vi "Follower SetControl.vi"(0 "DeviceReference":T1, 1 "StopSendingOtherRequests":bool=TRUE, 2 "MasterID":i32, 3 "OpposeMasterDirection":bool, 7 "error in":errorcluster, 18 "Update Frequency (Hz)":dbl=100.0) -> (20 "DeviceReference Out":T1, 27 "error out":errorcluster)   [LabVIEW 2023]
doc: "Follow the motor output of another Talon.\nIf Talon is in torque control, the torque is copied - which will increase the total torque applied. If Talon is in percent supply output control, the duty cycle is matched. Motor direction either matches master's configured direction or opposes it based on OpposeMasterDirection."
uses:
  Users/Cory/Documents/PhoenixPro-LabVIEW-Generation/controls/DeviceReference.ctl
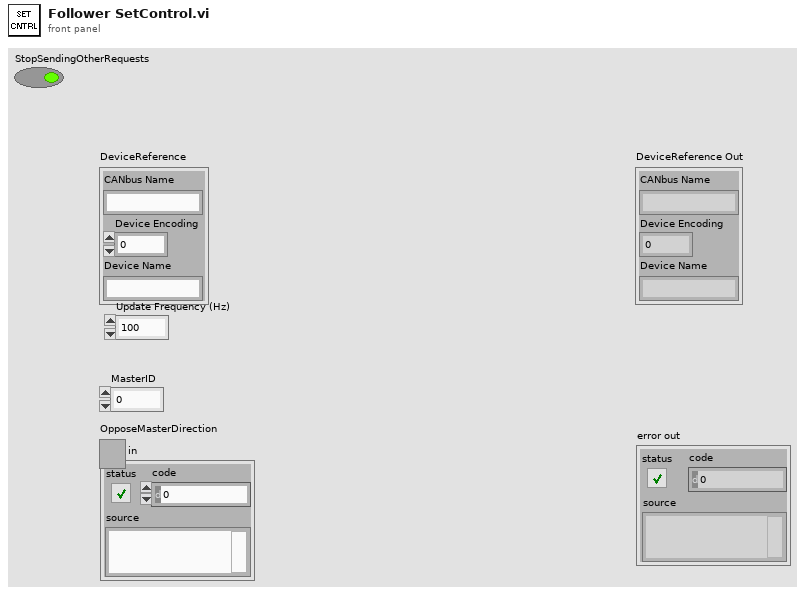
[diagram p1: front panel]
types:
  T1 = typedef "DeviceReference.ctl" = cluster{"CANbus Name":string, "Device Encoding":u32, "Device Name":string}
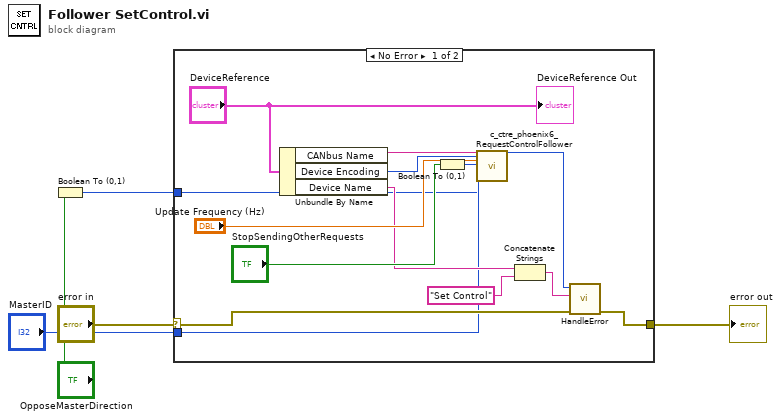
[diagram p0: block diagram]
diagram:
  n1 = Boolean To (0,1)(Boolean="OpposeMasterDirection") -> (0, 1=w1:i16)
  n2 = case shown="No Error" "error in" {
    selector: "error in" -> [w12 w20]
    tunnel: [w11 w20] -> w4
    tunnel: "MasterID" -> [w7 _]
    tunnel: w1 -> [w6 _]
    frame No Error {
      n3 = Unbundle By Name("DeviceReference") -> ("CANbus Name"=w18:string, "Device Encoding"=w17:u32, "Device Name"=w10:string)
      n4 = Boolean To (0,1)(Boolean="StopSendingOtherRequests") -> (0, 1=w14:i16)
      n5 = call <vilib>:"c_ctre_phoenix6_RequestControlFollower.vi"("String 2"=w18, "Numeric 2"=w17, "Numeric 3"="Update Frequency (Hz)", "Numeric 4"=w14, "Numeric 5"=w7, "Numeric 6"=w6) -> ("Numeric"=w13:i32)  [unwired: 20 in, 1 out]
      n6 = Concatenate Strings(w10, "Set Control" ("origin")) -> (w8:string)
      n7 = call "HandleError.vi"("error in"=w12, "origin"=w8, "Status"=w13) -> ("error out"=w11:errorcluster)  [unwired: 8 in]
      "DeviceReference Out" <- "DeviceReference"
    }
    frame Error {
    }
  }
  "error out" <- w4
